vi "RSZVB Configure Power Settings.vi"(7 "Fixed Power (-25.0)":dbl=-25.0 format="%^.3e", 8 "error in (no error)":errorcluster {"code" format="%.0x"}, 9 "Fundamental Power (0: RF)":i32(ring) items=["RF", "LO"], 10 "Channel (1)":i32=1, 11 "VISA session":refnum<visa-resource-name>) -> (0 "error out":errorcluster {"code" format="%.0x"}, 3 "dup VISA session":refnum<visa-resource-name>)   [LabVIEW 2011]
doc: "This VI configures the power settings for the mixer measurement.\n\nRemote-control command(s):\nSOURce<Ch>:]FREQuency:CONVersion:MIXer:FUNDamental RF | LO\nSOURce<Ch>:FREQuency:CONVersion:MIXer:PFIXed <fixed_power>"
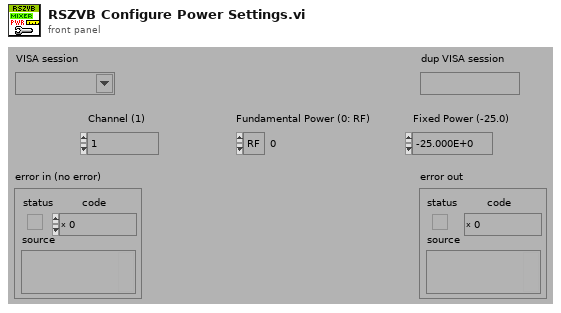
[diagram p1: front panel]
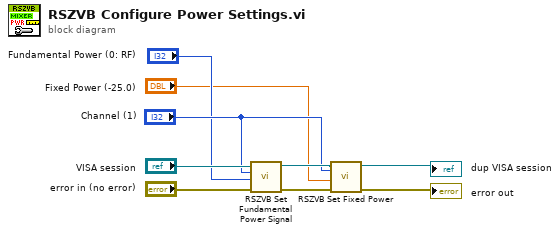
[diagram p0: block diagram]
diagram:
  n1 = call "RSZVB Set Fundamental Power Signal.vi"("error in (no error)"="error in (no error)", "Fundamental Power (0: RF)"="Fundamental Power (0: RF)", "Channel (1)"="Channel (1)", "VISA session"="VISA session") -> ("error out"=w5:errorcluster, "dup VISA session"=w8:refnum<visa-resource-name>)  [unwired: 6 in]
  n2 = call "RSZVB Set Fixed Power.vi"("error in (no error)"=w5, "Fixed Power (-25.0)"="Fixed Power (-25.0)", "Channel (1)"="Channel (1)", "VISA session"=w8) -> ("error out"=→"error out":errorcluster, "dup VISA session"=→"dup VISA session":refnum<visa-resource-name>)  [unwired: 6 in]
